vi "AlignDUTVariables.vi"() -> ()   [LabVIEW 2018]
uses:
  <vilib>/regexp/Match Regular Expression.xnode
panel:
  out "Y 4":dbl format="%#_8g"
  out "X 4":dbl format="%#_8g"
  out "error out":errorcluster
  out "Y 3":dbl format="%#_8g"
  out "X 3":dbl format="%#_8g"
  in  "error in (no error)":errorcluster
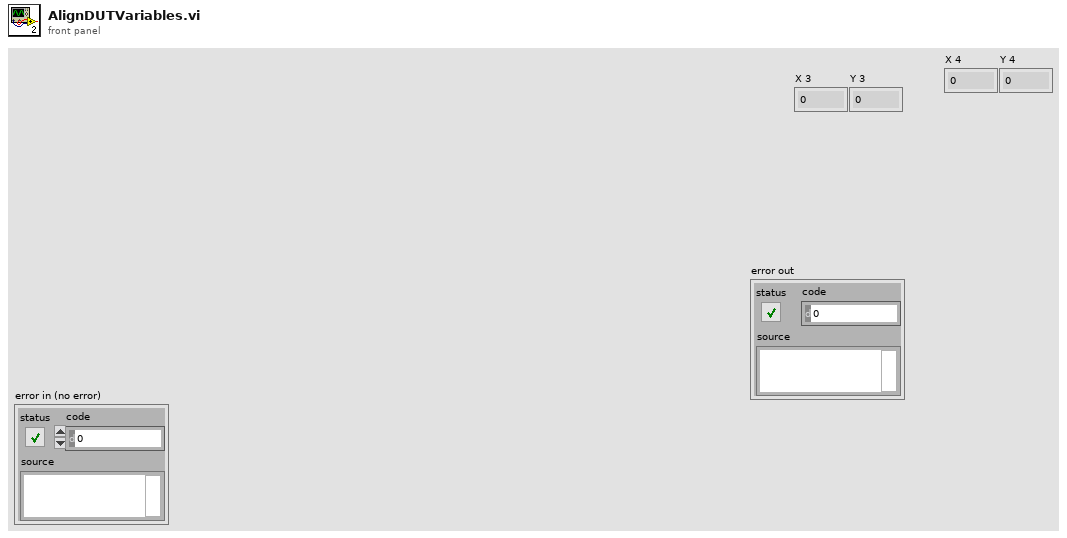
[diagram p1: front panel]
types:
  T1 = enum16{"Standard", "Buffered", "CRLF", "Immediate"}
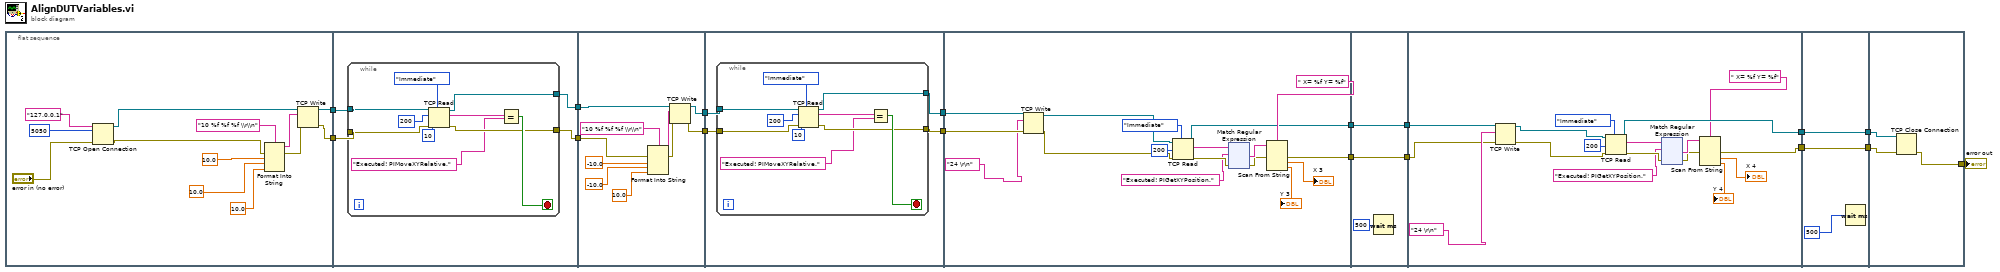
[diagram p0: block diagram]
diagram:
  n1 = flat-sequence {
    tunnel: [w19] -> w17
    tunnel: [w18] -> w16
    tunnel: w17 -> [w33]
    tunnel: w16 -> [w34]
    tunnel: [w32] -> w15
    tunnel: [w31] -> w14
    tunnel: w15 -> [w51]
    tunnel: w14 -> [w47]
    tunnel: [w46] -> w13
    tunnel: [w45] -> w12
    tunnel: w13 -> [w58]
    tunnel: w12 -> [w57]
    tunnel: [w55] -> w11
    tunnel: [w56] -> w10
    tunnel: w11 -> [w72]
    tunnel: w10 -> [w73]
    tunnel: [w75] -> w9
    tunnel: [w74] -> w8
    tunnel: w9 -> [w202]
    tunnel: w8 -> [w201]
    tunnel: [w202] -> w7
    tunnel: [w201] -> w6
    tunnel: w7 -> [w206]
    tunnel: w6 -> [w205]
    tunnel: [w210] -> w5
    tunnel: [w208] -> w1
    tunnel: w5 -> [w335]
    tunnel: [w336] -> w4
    tunnel: [w335] -> w3
    tunnel: w1 -> [w336]
    tunnel: w4 -> [w339]
    tunnel: w3 -> [w338]
    tunnel: [w337] -> w2
    frame #0 {
      n2 = TCP Open Connection(address="127.0.0.1", remote port or service name=u16 5050, error in (no error)="error in (no error)") -> (connection ID=w20:refnum<k5>, error out=w21:errorcluster)  [unwired: 2 in]
      n3 = Format Into String(format string="10 %f %f %f \\r\\n", error in=w21, 10.0 ("X"), 10.0 ("Y"), 10.0 ("input 3")) -> (resulting string=w23:string, error out=w22:errorcluster)  [unwired: 1 in]
      n4 = TCP Write(connection ID=w20, data in=w23, error in (no error)=w22) -> (connection ID out=w18:refnum<k5>, error out=w19:errorcluster)  [unwired: 1 in, 1 out]
    }
    frame #1 {
      n5 = while {
        tunnel: w34 -> [w42]
        tunnel: w33 -> [w41]
        tunnel: [w37] -> w32
        tunnel: [w36] -> w31
        stop <- w38 stop-if-true
        n6 = TCP Read(connection ID=w42, bytes to read=200, error in (no error)=w41, 7:T1."Immediate" ("mode (standard)"), 9:10 ("timeout ms (25000)")) -> (connection ID out=w36:refnum<k5>, data out=w39:string, error out=w37:errorcluster)
        n7 = Equal?(x=w39, y="Executed! PIMoveXYRelative.") -> (x = y?=w38:bool)
      }
    }
    frame #2 {
      n8 = Format Into String(format string="10 %f %f %f \\r\\n", error in=w51, -10.0 ("X 2"), -10.0 ("Y 2"), 10.0 ("input 3")) -> (resulting string=w53:string, error out=w54:errorcluster)  [unwired: 1 in]
      n9 = TCP Write(connection ID=w47, data in=w53, error in (no error)=w54) -> (connection ID out=w45:refnum<k5>, error out=w46:errorcluster)  [unwired: 1 in, 1 out]
    }
    frame #3 {
      n10 = while {
        tunnel: w58 -> [w66]
        tunnel: [w62] -> w55
        tunnel: [w61] -> w56
        tunnel: w57 -> [w59]
        stop <- w63 stop-if-true
        n11 = TCP Read(connection ID=w59, bytes to read=200, error in (no error)=w66, 7:T1."Immediate" ("mode (standard)"), 9:10 ("timeout ms (25000)")) -> (connection ID out=w61:refnum<k5>, data out=w64:string, error out=w62:errorcluster)
        n12 = Equal?(x=w64, y="Executed! PIMoveXYRelative.") -> (x = y?=w63:bool)
      }
    }
    frame #4 {
      n13 = TCP Write(connection ID=w73, data in="24 \r\n" ("initial string"), error in (no error)=w72) -> (connection ID out=w70:refnum<k5>, error out=w71:errorcluster)  [unwired: 1 in, 1 out]
      n14 = TCP Read(connection ID=w70, bytes to read=200, error in (no error)=w71, 7:T1."Immediate" ("mode (standard)")) -> (connection ID out=w74:refnum<k5>, data out=w82:string, error out=w83:errorcluster)  [unwired: 1 in]
      n15 = xnode "Match Regular Expression"("input string"=w82, "regular expression"="Executed! PIGetXYPosition.", "error in"=w83) -> ("after match"=w85:string, "error out"=w84:errorcluster)  [unwired: 3 in, 3 out]
      n16 = Scan From String(format string=" X= %f Y= %f", input string=w85, error in=w84) -> (error out=w75:errorcluster, output 1=→"X 3":dbl, output 2=→"Y 3":dbl)  [unwired: 3 in, 2 out]
    }
    frame #5 {
      n17 = Wait (ms)(milliseconds to wait=u32 500) -> ()  [unwired: 1 out]
    }
    frame #6 {
      n18 = TCP Write(connection ID=w205, data in="24 \r\n" ("initial string"), error in (no error)=w206) -> (connection ID out=w204:refnum<k5>, error out=w203:errorcluster)  [unwired: 1 in, 1 out]
      n19 = TCP Read(connection ID=w204, bytes to read=200, error in (no error)=w203, 7:T1."Immediate" ("mode (standard)")) -> (connection ID out=w210:refnum<k5>, data out=w216:string, error out=w217:errorcluster)  [unwired: 1 in]
      n20 = xnode "Match Regular Expression"("input string"=w216, "regular expression"="Executed! PIGetXYPosition.", "error in"=w217) -> ("after match"=w219:string, "error out"=w218:errorcluster)  [unwired: 3 in, 3 out]
      n21 = Scan From String(format string=" X= %f Y= %f", input string=w219, error in=w218) -> (error out=w208:errorcluster, output 1=→"X 4":dbl, output 2=→"Y 4":dbl)  [unwired: 3 in, 2 out]
    }
    frame #7 {
      n22 = Wait (ms)(milliseconds to wait=u32 500) -> ()  [unwired: 1 out]
    }
    frame #8 {
      n23 = TCP Close Connection(connection ID=w338, error in (no error)=w339) -> (error out=w337:errorcluster)  [unwired: 1 in, 1 out]
    }
  }
  "error out" <- w2
